vi "StartMotionAbsolute.vi"(8 "error in (no error)":errorcluster, 9 "Axis (1..4)":T1=1 items=["X"=1, "Y"=2, "Z"=3, "T"=4], 10 "Absolute Position, mm or deg.":dbl, 11 "VXMx2 in":refnum<class "VXMx2.lvclass">) -> (0 "error out":errorcluster, 3 "VXMx2 out":refnum<class "VXMx2.lvclass">)   [LabVIEW 2019, in "VXMx2.lvclass"]
uses:
  VXMx2.lvclass
  <instrlib>/Velmex VXM/Public/VXM Axis.ctl
  VXMx2.lvclass/VXMx2.ctl
  <instrlib>/Velmex VXM/Velmex VXM.lvlib
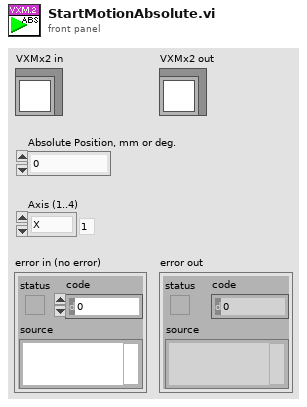
[diagram p1: front panel]
types:
  T1 = typedef "Velmex VXM.lvlib/VXM Axis.ctl" = u16
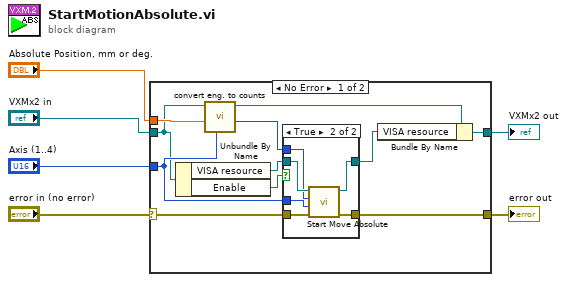
[diagram p0: block diagram]
diagram:
  n1 = case shown="No Error" "error in (no error)" {
    selector: "error in (no error)" -> [w14 w27]
    tunnel: [w13 w27] -> w5
    tunnel: [w17 w26] -> w3
    tunnel: "VXMx2 in" -> [w8 w26]
    tunnel: "Absolute Position, mm or deg." -> [w11 _]
    tunnel: "Axis (1..4)" -> [w9 _]
    frame No Error {
      n2 = Unbundle By Name(w8) -> ("VISA resource"=w16:refnum<visa-resource-name>, "Enable"=w12:bool)
      n3 = call "convert eng. to counts.vi"("Axis (1..4)"=w9, "Position, eng units"=w11, "VXMx2 in"=w8) -> ("Position, counts"=w10:i32, "VXMx2 out"=w7:refnum<class "VXMx2.lvclass">)  [unwired: 5 in, 2 out]
      n4 = case shown="True" w12 {
        tunnel: w16 -> [w19 w25]
        tunnel: [w19 w24] -> w15
        tunnel: w14 -> [w18 w23]
        tunnel: [w18 w22] -> w13
        tunnel: w10 -> [_ w21]
        tunnel: w9 -> [_ w20]
        frame False {
        }
        frame True {
          n5 = call <instrlib>:"Start Move Absolute.vi"("error in (no error)"=w23, "Axis (1..4)"=w20, "Absolute Position, counts"=w21, "VISA resource name"=w25) -> ("error out"=w22:errorcluster, "VISA resource out"=w24:refnum<visa-resource-name>)  [unwired: 6 in]
        }
      }
      n6 = Bundle By Name(cluster=w7, "VISA resource"=w15) -> (w17:refnum<class "VXMx2.lvclass">)
    }
    frame Error {
    }
  }
  "error out" <- w5
  "VXMx2 out" <- w3
